vi "精简框图1.vi"(0 "mid_str_labelType":string="None", 1 "mid_array_eep":string[][](array[string])=[["11", "11", "0", "0"], ["7", "0", "0", "0"], ["2", "23", "0", "0"], ["0", "80", "0", "0"], ["0", "0", "0", "0"], ["0", "0", "0", "0"], ["0", "0", "0", "0"], ["0", "0", "0", "0"], ["0", "0", "0", "0"], ["0", "80", "0", "0"], ["0", "0", "0", "0"], ["0", "0", "0", "0"], ["0", "FF", "0", "0"], ["0", "0", "0", "0"], ["0", "0", "0", "0"], ["0", "0", "0", "0"], ["0", "0", "0", "0"], ["0", "0", "0", "0"], ["0", "1", "0", "0"], ["0", "A0", "0", "0"], ["0", "4C", "0", "0"], ["0", "55", "0", "0"], ["0", "58", "0", "0"], ["0", "53", "0", "0"], ["0", "48", "0", "0"], ["0", "41", "0", "0"], ["0", "52", "0", "0"], ["0", "45", "0", "0"], ["0", "2D", "0", "0"], ["0", "49", "0", "0"], ["0", "43", "0", "0"], ["0", "54", "0", "0"], ["0", "20", "0", "0"], ["0", "20", "0", "0"], ["0", "20", "0", "0"], ["0", "20", "0", "0"], ["0", "1F", "0", "0"], ["0", "3C", "0", "0"], ["0", "18", "0", "0"], ["0", "A0", "0", "0"], ["0", "48", "0", "0"], ["0", "48", "0", "0"], ["0", "33", "0", "0"], ["0", "43", "0", "0"], ["0", "30", "0", "0"], ["0", "34", "0", "0"], ["0", "30", "0", "0"], ["0", "34", "0", "0"], ["0", "57", "0", "0"], ["0", "34", "0", "0"], ["0", "31", "0", "0"], ["0", "33", "0", "0"], ["0", "57", "0", "0"], ["0", "58", "0", "0"], ["0", "20", "0", "0"], ["0", "20", "0", "0"], ["0", "41", "0", "0"], ["0", "20", "0", "0"], ["0", "3", "0", "0"], ["0", "4", "0", "0"], ["0", "5", "0", "0"], ["0", "8", "0", "0"], ["0", "46", "0", "0"], ["0", "47", "0", "0"], ["0", "B", "0", "0"], ["0", "0", "0", "0"], ["0", "0", "0", "0"], ["0", "0", "0", "0"], ["0", "31", "0", "0"], ["0", "35", "0", "0"], ["0", "32", "0", "0"], ["0", "32", "0", "0"], ["0", "34", "0", "0"], ["0", "34", "0", "0"], ["0", "30", "0", "0"], ["0", "30", "0", "0"], ["0", "35", "0", "0"], ["0", "20", "0", "0"], ["0", "20", "0", "0"], ["0", "20", "0", "0"], ["0", "20", "0", "0"], ["0", "20", "0", "0"], ["0", "20", "0", "0"], ["0", "20", "0", "0"], ["0", "31", "0", "0"], ["0", "35", "0", "0"], ["0", "30", "0", "0"], ["0", "39", "0", "0"], ["0", "30", "0", "0"], ["0", "31", "0", "0"], ["0", "20", "0", "0"], ["0", "20", "0", "0"], ["0", "0", "0", "0"], ["0", "0", "0", "0"], ["0", "67", "0", "0"], ["0", "89", "0", "0"], ["0", "0", "0", "0"], ["0", "0", "0", "0"], ["0", "0", "0", "0"], ["0", "0", "0", "0"], ["0", "0", "0", "0"], ["0", "0", "0", "0"], ["0", "0", "0", "0"], ["0", "0", "0", "0"], ["0", "0", "0", "0"], ["0", "0", "0", "0"], ["0", "0", "0", "0"], ["0", "0", "0", "0"], ["0", "0", "0", "0"], ["0", "0", "0", "0"], ["0", "0", "0", "0"], ["0", "0", "0", "0"], ["0", "0", "0", "0"], ["0", "0", "0", "0"], ["0", "0", "0", "0"], ["0", "0", "0", "0"], ["0", "0", "0", "0"], ["0", "0", "0", "0"], ["0", "0", "0", "0"], ["0", "0", "0", "0"], ["0", "0", "0", "0"], ["0", "0", "0", "0"], ["0", "0", "0", "0"], ["0", "0", "0", "0"], ["0", "0", "0", "0"], ["0", "0", "0", "0"], ["0", "0", "0", "0"], ["0", "0", "0", "0"]], 2 "mid_str_snformat":string, 3 "Convert Style":bool, 4 "DateCode8Value_0X30":dbl, 5 "P/N":string, 7 "Sart SN":i32, 9 "校验信息":T1(array[cluster])) -> (13 "LocalSN Generate Status":string, 14 "midVar_time_date":timestamp=timestamp(3527207877 s since 1904-01-01), 15 "midVar_str_SN":string, 16 "mid_array_temp_int":u8[][](array[numeric])=[[3, 4, 33, 0, 0, 0, 0, 65, 4, 128, 213, 0, 103, 0, 0, 0, 0, 0, 0, 0, 0, 0, 0, 0, 0, 0, 0, 0, 0, 0, 0, 0, 0, 0, 0, 0, 0, 0, 0, 0, 0, 0, 0, 0, 0, 0, 0, 0, 0, 0, 0, 0, 0, 0, 0, 0, 0, 0, 0, 0, 1, 0, 0, 42, 0, 0, 0, 0, 0, 0, 0, 0, 0, 0, 0, 0, 0, 0, 0, 0, 0, 0, 0, 0, 49, 52, 49, 49, 50, 53, 0, 0, 0, 0, 0, 46, 0, 0, 0, 0, 0, 0, 0, 0, 0, 0, 0, 0, 0, 0, 0, 0, 0, 0, 0, 0, 0, 0, 0, 0, 0, 0, 0, 0, 0, 0, 0, 0, 0, 0, 0, 0, 0, 0, 0, 0, 0, 0, 0, 0, 0, 0, 0, 0, 0, 0, 0, 0, 0, 0, 0, 0, 0, 0, 0, 0, 0, 0, 0, 0, 0, 0, 0, 0, 0, 0, 0, 0, 0, 0, 0, 0, 0, 0, 0, 0, 0, 0, 0, 0, 0, 0, 0, 0, 0, 0, 0, 0, 0, 0, 0, 0, 0, 0, 0, 0, 0, 0, 0, 0, 0, 0, 0, 0, 0, 0, 0, 0, 0, 0, 0, 0, 0, 0, 0, 0, 0, 0, 0, 0, 0, 0, 0, 0, 0, 0, 0, 0, 0, 0, 0, 0, 0, 0, 0, 0, 0, 0, 0, 0, 0, 0, 0, 0, 0, 0, 0, 0, 0, 0, 0, 0, 0, 0, 0, 0]] format="%.0x", 17 "S/N:":string="153410001", 18 "Report No.":string="HF-153410001", 19 "Sample #":string="153410001")   [LabVIEW 2011]
panel:
  # "读取labelType中的客户信息"
  # "SN的格式信息"
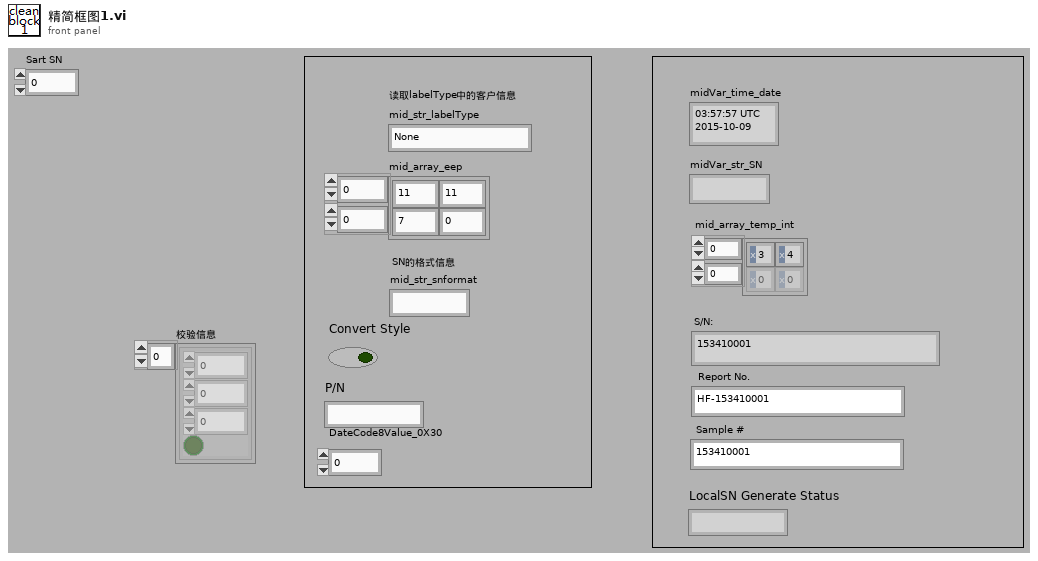
[diagram p1: front panel]
types:
  T1 = cluster{"start":i32, "length":i32, "p":i32, "H/L":bool}[]
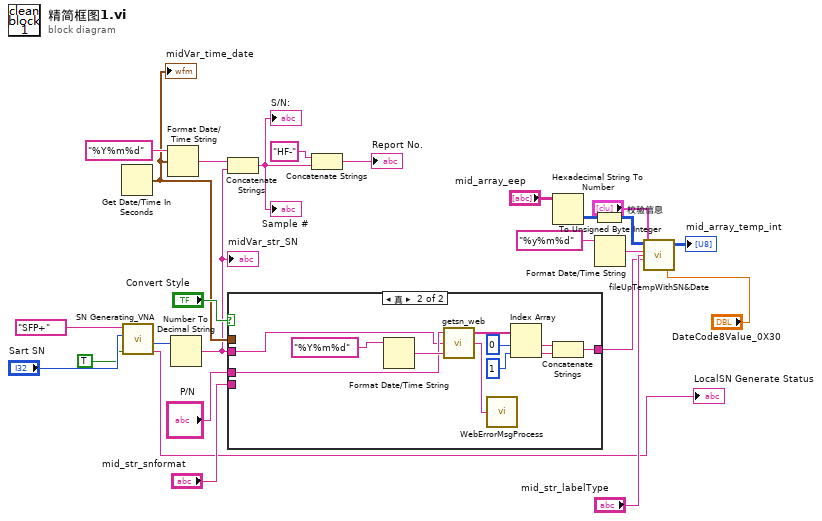
[diagram p0: block diagram]
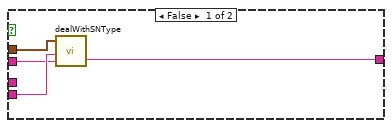
[diagram p2: hidden frame]
diagram:
  n1 = Get Date/Time In Seconds() -> (seconds since 1Jan1904=w8:timestamp)
  "midVar_time_date" <- w8
  n2 = call "SN Generating_VNA.vi"("Start"=TRUE, "Sart SN"="Sart SN", "Product Type"="SFP+") -> ("note"=→"LocalSN Generate Status":string, "show_int_XXXX"=w22:i32)  [unwired: 2 in, 2 out]
  n3 = Format Date/Time String(time format string (%c)="%Y%m%d" ("时间格式字符串(%c)"), seconds (now)=w8) -> (date/time string=w20:string)  [unwired: 1 in]
  n4 = Number To Decimal String(number=w22) -> (decimal integer string=w6:string)  [unwired: 1 in]
  "midVar_str_SN" <- w6
  n5 = Concatenate Strings(w20, w6) -> (w10:string)
  "S/N:" <- w10
  "Sample #" <- w10
  n6 = case shown="真" "Convert Style" {
    tunnel: [w29 w34] -> w5
    tunnel: w8 -> [w28 _]
    tunnel: "mid_str_snformat" -> [w27 _]
    tunnel: w6 -> [w26 w30]
    tunnel: "P/N" -> [_ w31]
    frame False {
      n7 = call "dealWithSNType.vi"("SNXn"=w26, "SNType"=w27, "TimeInput"=w28) -> ("show_str_SNwithWholeFormat"=w29:string)  [unwired: 1 out]
    }
    frame True {
      n8 = Format Date/Time String(time format string (%c)="%Y%m%d" ("时间格式字符串(%c)")) -> (date/time string=w32:string)  [unwired: 2 in]
      n9 = call "getsn_web.vi"("strDate"=w32, "sSN"=w30, "strPartNo"=w31) -> ("strErrMsg"=w40:string, "getCode"=w39:string[])  [unwired: 1 out]
      n10 = call "WebErrorMsgProcess.vi"("WebErrorMsg"=w40) -> ()
      n11 = Index Array(array=w39, index #1=0 ("索引"), index #2=1 ("索引")) -> (element #1=w36:string, element #2=w35:string)
      n12 = Concatenate Strings(w36, w35) -> (w34:string)
    }
  }
  n13 = Concatenate Strings("HF-" ("字符串"), w10) -> (→"Report No.":string)
  n14 = Hexadecimal String To Number(string="mid_array_eep") -> (number=w18:u32[][])  [unwired: 2 in, 1 out]
  n15 = To Unsigned Byte Integer(number=w18) -> (unsigned 8bit integer=w17:u8[][])
  n16 = Format Date/Time String(time format string (%c)="%y%m%d" ("时间格式字符串(%c)")) -> (date/time string=w15:string)  [unwired: 2 in]
  n17 = call "fileUpTempWithSN&Date.vi"("input_array_temp_int"=w17, "input_str_Date"=w15, "input_str_SN"=w5, "校验信息"="校验信息", "input_str_customer"="mid_str_labelType", "DateCode8Value_0X30"="DateCode8Value_0X30") -> ("show_array_temp_int"=→"mid_array_temp_int":u8[][])  [unwired: 1 out]
